vi "Functional Imaging-Z-plane selection management.vi"(8 "error in":errorcluster) -> (0 "error out":errorcluster, 1 "GreenPOIMax":T1, 3 "RedPOIMax":T1)   [LabVIEW 2020]
uses:
  <vilib>/vision/Image Controls.llb/IMAQ Image.ctl
  Typedefs/Get-Set-Clear Control.ctl
  Typedefs/ROI parameters data type.ctl
  Global variables/gl_Functional Imaging-Global variables.vi
  <vilib>/vision/NI_Vision_Development_Module.lvlib
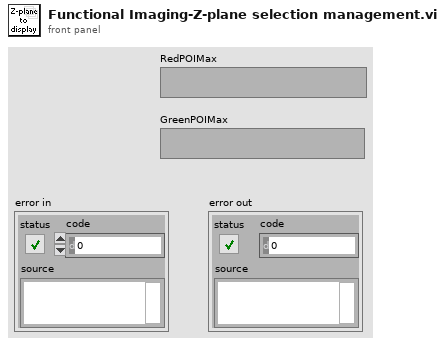
[diagram p1: front panel]
types:
  T1 = typedef "IMAQ Image.ctl" = refnum<image>
  T2 = typedef "Get-Set-Clear Control.ctl" = enum16{"Get", "Set", "Clear"}
  T3 = typedef "Functional Imging UI Refs.ctl" = cluster{"Menu ref":refnum<k9>, "Image control":refnum<vi>, "VI ref":refnum<vi>, "XGrapher":refnum<vi>, "Smoothing":refnum<vi>, "POI Averaging":refnum<vi>, "Normalize":refnum<vi>, "POI data points in each trial":refnum<vi>, "Channel":refnum<vi>, "Experiment data folder path":refnum<vi>, "[ROI vis]":refnum<vi>, "[Groups] visbl":T4, "Group Name":refnum<vi>, "POI index":refnum<vi>, "Trial No.":refnum<vi>, "Intensity Zoom":refnum<vi>, "Trial Cursor Enabled":refnum<vi>, "Number of Trials (ind 1)":refnum<vi>, "Number of Trials (ind 2)":refnum<vi>, "MiniScans Available":refnum<vi>, "POI Available":refnum<vi>, "Defer graph updates":refnum<vi>, "Waveform selector":refnum<vi>, "#of selected POI":refnum<vi>, "#of selected MiniScans":refnum<vi>, "#of selected groups":refnum<vi>, "Max Z-Projection":refnum<vi>, "Z-Plane Selector":refnum<vi>, "Index of miniscan point to visualise":refnum<vi>, "ROI vis. mode":refnum<vi>, "Total # of points":refnum<vi>, "Index of group clicked on":refnum<vi>, "Pane 1":refnum<vi>, "Pane 2":refnum<vi>, "Pane 3":refnum<vi>, "Pane 4":refnum<vi>, "Pane 5":refnum<vi>, "Pane 6":refnum<vi>, "Deselect all ROI":refnum<vi>, "Deselect all groups":refnum<vi>}
  T4 = typedef "Groups array referecne.ctl" = refnum<vi>
  T5 = enum32{"Average", "Min", "Max", "Clear  if < ", "Clear  if < or =", "Clear  if =", "Clear  if > or =", "Clear  if >"}
  T6 = typedef "ROI parameters data type.ctl" = cluster{"ROI index":dbl, "ROI ID":dbl, "ROI Time (ns)":dbl, "Pixels in ROI":dbl, "X start":dbl, "Y start":dbl, "Z start":dbl, "X stop":dbl, "Y stop":dbl, "Z stop":dbl, "Angle (deg)":dbl, "Composite ID":dbl, "Number of lines":dbl, "Frame Size":dbl, "Zoom":dbl, "Laser Power (%)":dbl, "ROI group ID":dbl, "Resolution":dbl, "Dwell Time per pixel":dbl, "Pixels per miniscan":dbl, "Original FOV (um)":dbl, "Apparent Frame Size":dbl, "Z Plane Idx":i32[], "Z Plane codes":i32[]}
  T7 = typedef "Image Type" = u32
  T8 = typedef "ROI visibility mode.ctl" = enum16{"Show all ROI when scrolling in Z", "Show only selected ROI when scrolling in Z"}
  T9 = typedef "ROI selector array-ROI vis.ctl" = T10[]
  T10 = typedef "Interface-ROI selection cluster.ctl" = cluster{"ROI number":i32, "ROI ID":T11, "Visibility":bool}
  T11 = typedef "ROI ID Enum.ctl" = enum16{"Point", "MiniScan", "Comp. MiniScan", "Rectangle", "Comp. volume", "Arb. plane point", "None"}
  T12 = typedef "Functional Parameters Cluster.ctl" = cluster{"ROI data":dbl[][], "ROI format version":i32, "Norm ROI data":dbl[][], "Norm. ROI format version":i32, "Z norm":dbl[], "Z norm format version":i32}
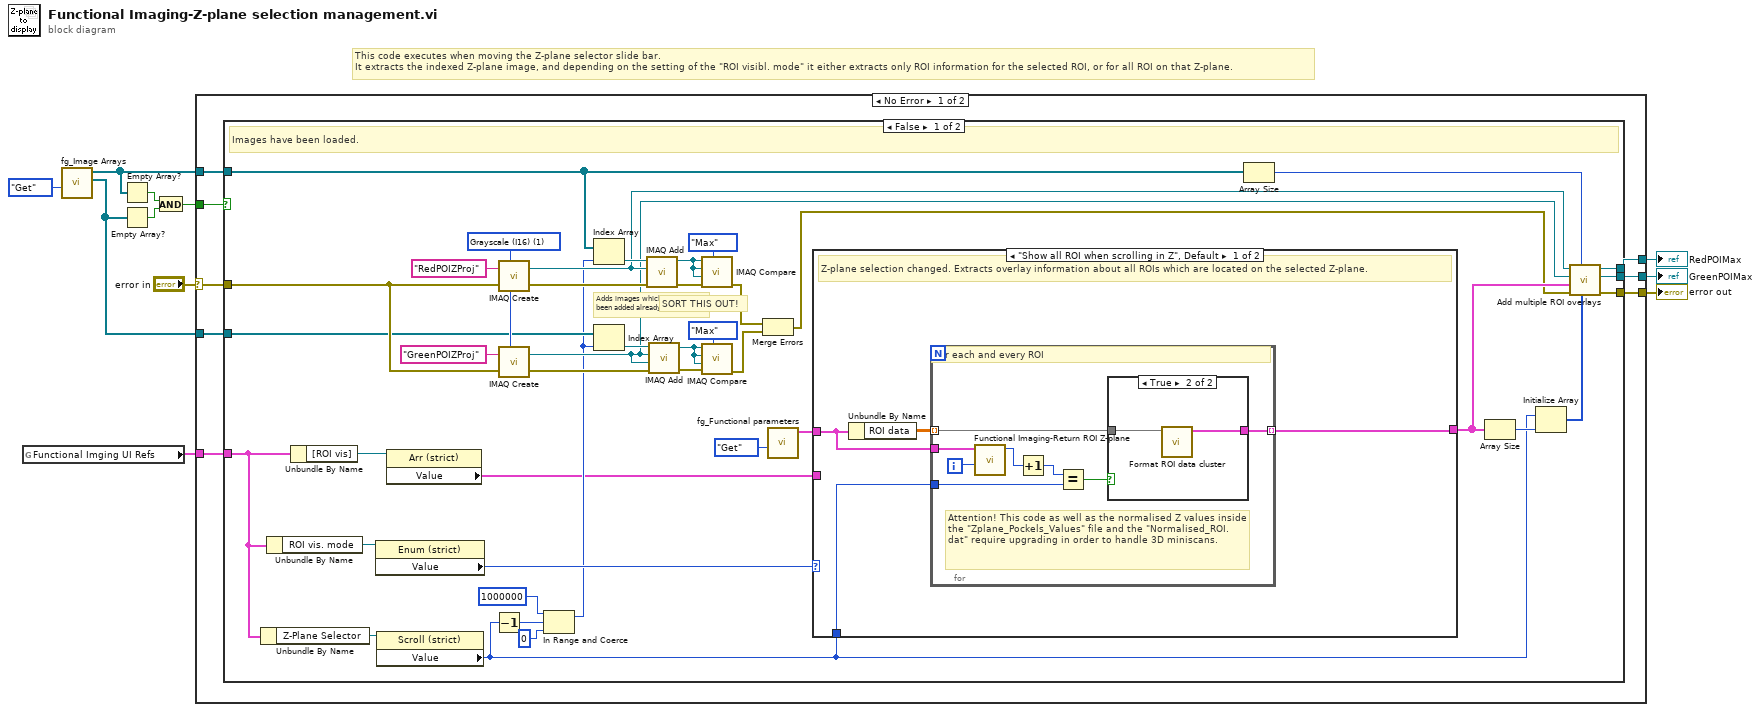
[diagram p0: block diagram]
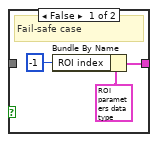
[diagram p2: hidden frame]
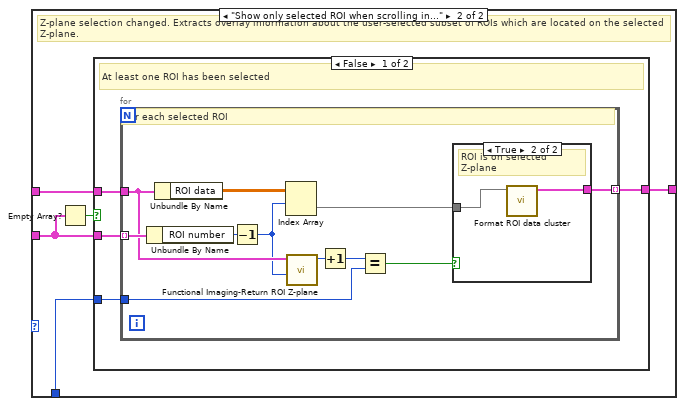
[diagram p3: hidden frame]
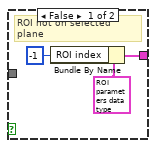
[diagram p4: hidden frame]
diagram:
  # "This code executes when moving the Z-plane selector slide bar.\nIt extracts the indexed Z-plane image, and depending on the setting of the \"ROI visibl. mode\" it either extracts only ROI information for the selected ROI, or for all ROI on that Z-plane."
  n1 = global read "gl_Functional Imaging-Global variables.vi" "Functional Imging UI Refs"() -> (w1:T3)
  n2 = call "fg_Image Arrays.vi"("Function"=Get-Set-Clear_Control."Get") -> ("Green Images Array"=w3:T1[], "Red Images Array"=w4:T1[])  [unwired: 9 in]
  n3 = Empty Array?(array=w4) -> (empty?=w6:bool)
  n4 = Empty Array?(array=w3) -> (empty?=w7:bool)
  n5 = And(x=w6, y=w7) -> (x .and. y?=w2:bool)
  n6 = case shown="No Error" "error in" {
    selector: "error in" -> [w16 w103]
    tunnel: [w17 _] -> w11
    tunnel: [w18 _] -> w10
    tunnel: [w19 w103] -> w9
    tunnel: w1 -> [w15 _]
    tunnel: w4 -> [w14 _]
    tunnel: w3 -> [w13 _]
    tunnel: w2 -> [w12 _]
    frame No Error {
      n7 = case shown="False" w12 {
        tunnel: [w55 _] -> w19
        tunnel: [w54 _] -> w18
        tunnel: [w53 _] -> w17
        tunnel: w16 -> [w52 _]
        tunnel: w15 -> [w34 _]
        tunnel: w14 -> [w27 _]
        tunnel: w13 -> [w26 _]
        frame False {
          w60 = T7 1 items=["Grayscale (U8)", "Grayscale (I16)", "Grayscale (SGL)", "Complex (CSG)", "RGB (U32)", "HSL (U32)", "RGB (U64)"] ("Image Type")
          # "SORT THIS OUT!"
          # "Adds images which have not\nbeen added already."
          # "Images have been loaded."
          n8 = Unbundle By Name(w34) -> ("Z-Plane Selector"=w48:refnum<vi>)
          n9 = Unbundle By Name(w34) -> ("ROI vis. mode"=w35:refnum<vi>)
          n10 = Unbundle By Name(w34) -> ("[ROI vis]"=w49:refnum<vi>)
          n11 = property on="Property Node" class="Enum (strict)"(reference=w35) -> ("Value"=w33:T8)  [unwired: 1 in, 2 out]
          n12 = property on="Property Node" class="Scroll (strict)"(reference=w48) -> ("Value"=w25:i32)  [unwired: 1 in, 2 out]
          n13 = property on="Property Node" class="Arr (strict)"(reference=w49) -> ("Value"=w20:T9)  [unwired: 1 in, 2 out]
          n14 = Decrement(x=w25) -> (x-1=w24:i32)
          n15 = call "IMAQ Create"("Image Name"="RedPOIZProj" ("string"), "Image Type"=w60, "error in (no error)"=w52) -> ("New Image"=w32:T1, "error out"=w56:errorcluster)  [unwired: 2 in]
          n16 = call "IMAQ Create"("Image Name"="GreenPOIZProj" ("string"), "Image Type"=w60, "error in (no error)"=w52) -> ("New Image"=w31:T1, "error out"=w57:errorcluster)  [unwired: 2 in]
          n17 = In Range and Coerce(upper limit=1000000, x=w24, lower limit=0) -> (coerced(x)=w23:i32)  [unwired: 1 out]
          n18 = Index Array(array=w27, index=w23) -> (element=w41:T1)
          n19 = Index Array(array=w26, index=w23) -> (element=w45:T1)
          n20 = call "IMAQ Add"("Image Src A"=w41, "Image Dst"=w32, "error in (no error)"=w56) -> ("Image Dst Out"=w40:T1, "error out"=w43:errorcluster)  [unwired: 4 in]
          n21 = call "IMAQ Add"("Image Src A"=w45, "Image Dst"=w31, "Image Src B"=w31, "error in (no error)"=w57) -> ("Image Dst Out"=w44:T1, "error out"=w42:errorcluster)  [unwired: 3 in]
          n22 = call "IMAQ Compare"("Operator"=T5."Max", "error in (no error)"=w43, "Image Src B"=w40, "Image Dst"=w40, "Image Src A"=w40) -> ("error out"=w29:errorcluster)  [unwired: 5 in, 1 out]
          n23 = call "IMAQ Compare"("Operator"=T5."Max", "error in (no error)"=w42, "Image Src B"=w44, "Image Dst"=w44, "Image Src A"=w44) -> ("error out"=w30:errorcluster)  [unwired: 5 in, 1 out]
          n24 = Merge Errors(w29, w30) -> (w28:errorcluster)
          n25 = call "fg_Functional parameters.vi"("Function"=Get-Set-Clear_Control."Get") -> ("Functional Parameters"=w50:T12)  [unwired: 7 in, 3 out]
          n26 = case shown="\"Show all ROI when scrolling in Z\", Default" w33 {
            tunnel: w50 -> [w63 w82]
            tunnel: w25 -> [w61 w81]
            tunnel: [w62 w80] -> w38
            tunnel: w20 -> [_ w79]
            frame "Show all ROI when scrolling in Z", Default {
              # "Z-plane selection changed. Extracts overlay information about all ROIs which are located on the selected Z-plane."
              n27 = Unbundle By Name(w63) -> ("ROI data"=w64:dbl[][])
              n28 = for {
                tunnel: [w72] -> w62 mode=indexing
                tunnel: w64 -> [w70] mode=indexing
                tunnel: w63 -> [w71]
                tunnel: w61 -> [w66]
                i -> [w69]
                # "Attention! This code as well as the normalised Z values inside the \"Zplane_Pockels_Values\" file and the \"Normalised_ROI.dat\" require upgrading in order to handle 3D miniscans."
                # "For each and every ROI"
                n29 = call "Functional Imaging-Return ROI Z-plane.vi"("ROI index (zero based)"=w69, "Functional Parameters"=w71) -> ("Zero-based index of the Z-plane the indexed ROI belongs to"=w67:i32)  [unwired: 9 in]
                n30 = Increment(x=w67) -> (x+1=w68:i32)
                n31 = Equal?(x=w68, y=w66) -> (x = y?=w65:bool)
                n32 = case shown="True" w65 {
                  tunnel: w70 -> [_ w77]
                  tunnel: [w73 w76] -> w72
                  frame False {
                    # "Fail-safe case"
                    n33 = Bundle By Name(cluster=T6 {"ROI index"=0.0, "ROI ID"=0.0, "ROI Time (ns)"=0.0, "Pixels in ROI"=0.0, "X start"=0.0, "Y start"=0.0, "Z start"=0.0, "X stop"=0.0, "Y stop"=0.0, "Z stop"=0.0, "Angle (deg)"=0.0, "Composite ID"=0.0, "Number of lines"=0.0, "Frame Size"=0.0, "Zoom"=0.0, "Laser Power (%)"=0.0, "ROI group ID"=0.0, "Resolution"=0.0, "Dwell Time per pixel"=0.0, "Pixels per miniscan"=0.0, "Original FOV (um)"=0.0, "Apparent Frame Size"=0.0, "Z Plane Idx"=[], "Z Plane codes"=[]} ("X-Y-Z coordinates"), "ROI index"=i64 -1) -> (w73:T6)
                  }
                  frame True {
                    n34 = call "Format ROI data cluster.vi"("Single ROI info"=w77) -> ("X-Y-Z coordinates"=w76:T6)  [unwired: 10 in]
                  }
                }
              }
            }
            frame "Show only selected ROI when scrolling in Z" {
              # "Z-plane selection changed. Extracts overlay information about the user-selected subset of ROIs which are located on the selected Z-plane."
              n35 = Empty Array?(array=w79) -> (empty?=w78:bool)
              n36 = case shown="False" w78 {
                tunnel: w82 -> [w86 _]
                tunnel: w81 -> [w85 _]
                tunnel: [w84 _] -> w80
                tunnel: w79 -> [w83 _]
                frame False {
                  # "At least one ROI has been selected"
                  n37 = for {
                    tunnel: w83 -> [w97] mode=indexing
                    tunnel: [w90] -> w84 mode=indexing
                    tunnel: w86 -> [w89]
                    tunnel: w85 -> [w93]
                    # "For each selected ROI"
                    n38 = Unbundle By Name(w97) -> ("ROI number"=w95:i32)
                    n39 = Unbundle By Name(w89) -> ("ROI data"=w96:dbl[][])
                    n40 = Decrement(x=w95) -> (x-1=w88:i32)
                    n41 = Index Array(array=w96, index (row)=w88) -> (element=w91:dbl[])  [unwired: 1 in]
                    n42 = call "Functional Imaging-Return ROI Z-plane.vi"("ROI index (zero based)"=w88, "Functional Parameters"=w89) -> ("Zero-based index of the Z-plane the indexed ROI belongs to"=w87:i32)  [unwired: 9 in]
                    n43 = Increment(x=w87) -> (x+1=w94:i32)
                    n44 = Equal?(x=w94, y=w93) -> (x = y?=w92:bool)
                    n45 = case shown="True" w92 {
                      tunnel: w91 -> [_ w101]
                      tunnel: [w98 w102] -> w90
                      frame False {
                        # "ROI not on selected plane"
                        n46 = Bundle By Name(cluster=T6 {"ROI index"=0.0, "ROI ID"=0.0, "ROI Time (ns)"=0.0, "Pixels in ROI"=0.0, "X start"=0.0, "Y start"=0.0, "Z start"=0.0, "X stop"=0.0, "Y stop"=0.0, "Z stop"=0.0, "Angle (deg)"=0.0, "Composite ID"=0.0, "Number of lines"=0.0, "Frame Size"=0.0, "Zoom"=0.0, "Laser Power (%)"=0.0, "ROI group ID"=0.0, "Resolution"=0.0, "Dwell Time per pixel"=0.0, "Pixels per miniscan"=0.0, "Original FOV (um)"=0.0, "Apparent Frame Size"=0.0, "Z Plane Idx"=[], "Z Plane codes"=[]} ("X-Y-Z coordinates"), "ROI index"=i64 -1) -> (w98:T6)
                      }
                      frame True {
                        # "ROI is on selected Z-plane"
                        n47 = call "Format ROI data cluster.vi"("Single ROI info"=w101) -> ("X-Y-Z coordinates"=w102:T6)  [unwired: 10 in]
                      }
                    }
                  }
                }
                frame True {
                  # "No ROI selected"
                }
              }
            }
          }
          n48 = Array Size(array=w27) -> (size(s)=w39:i32)
          n49 = Array Size(array=w38) -> (size(s)=w37:i32)
          n50 = Initialize Array(w25, w37) -> (w36:i32[])
          n51 = call "Add multiple ROI overlays.vi"("[ROI index] (unity based)"=w36, "# of Z-planes"=w39, "error in"=w28, "[ROI info]"=w38, "Image 2 in"=w31, "Image 1 in"=w32) -> ("error out"=w55:errorcluster, "Image 2 out"=w53:T1, "Image 1 out"=w54:T1)  [unwired: 3 in]
        }
        frame True {
          # "No images loaded."
        }
      }
    }
    frame Error {
    }
  }
  "GreenPOIMax" <- w11
  "RedPOIMax" <- w10
  "error out" <- w9
